vi "Aircraft 2 Waypoints.vi"(7 "Method":enum16{"Get", "Set"}(ring), 11 "Waypoints In":T1[](array[typedef])) -> (3 "Waypoints Out":T1[](array[typedef]))   [LabVIEW 2014]
uses:
  MAVLink/Controls/Mission Planning Controls/MAVLINK Mission Item.ctl
  MAVLink/Controls/MAVLINK Mav Frame.ctl
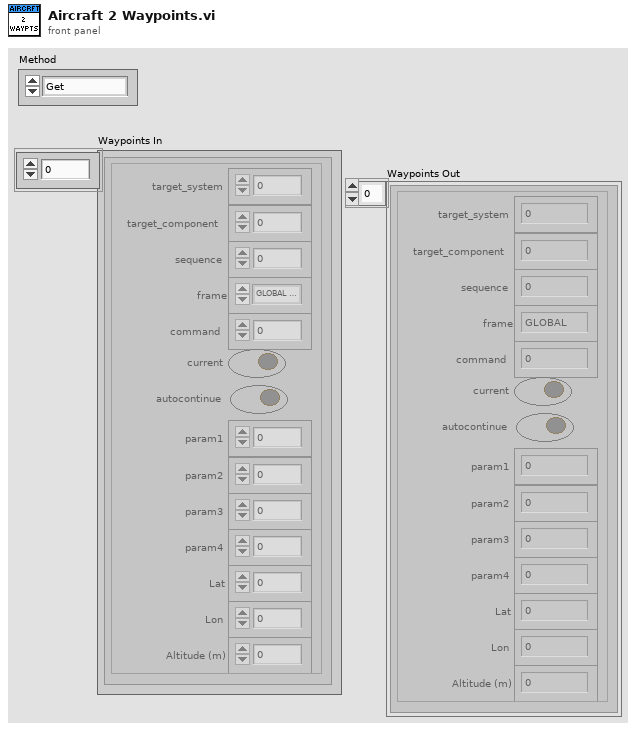
[diagram p1: front panel]
types:
  T1 = typedef "MAVLINK Mission Item.ctl" = cluster{"target_system":u8, "target_component":u8, "sequence":u16, "frame":T2, "command":u16, "current":bool, "autocontinue":bool, "param1":sgl, "param2":sgl, "param3":sgl, "param4":sgl, "Lat":sgl, "Lon":sgl, "Altitude (m)":sgl}
  T2 = typedef "MAVLINK Mav Frame.ctl" = enum8{"GLOBAL", "LOCAL NED", "MISSION", "GLOBAL RELATIVE ALT", "LOCAL ENU", "GLOBAL INT", "GLOBAL RELATIVE ALT INT", "LOCAL OFFSET NED", "BODY NED", "BODY OFFSET NED", "GLOBAL TERRAIN ALT", "GLOBAL TERRAIN ALT INT"}
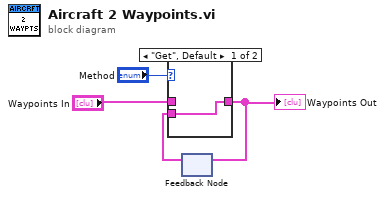
[diagram p0: block diagram]
diagram:
  n1 = feedback #1() -> (w2:T1[])  [unwired: 1 in]
  n2 = case shown="\"Get\", Default" "Method" {
    tunnel: "Waypoints In" -> [_ w6]
    tunnel: [w5 w6] -> w3
    tunnel: w2 -> [w5 _]
    frame "Get", Default {
    }
    frame "Set" {
    }
  }
  "Waypoints Out" <- w3
  n3 = feedback-in #1(w3) -> ()
